vi "Unsubscribe Client.vi"(8 "error in":errorcluster, 9 "Client":string, 10 "Topic Name":string, 11 "Broker in":refnum<class "Broker.lvclass">) -> (0 "error out":errorcluster, 3 "Broker out":refnum<class "Broker.lvclass">)   [LabVIEW 2014, in "Broker.lvclass"]
uses:
  Broker.lvclass
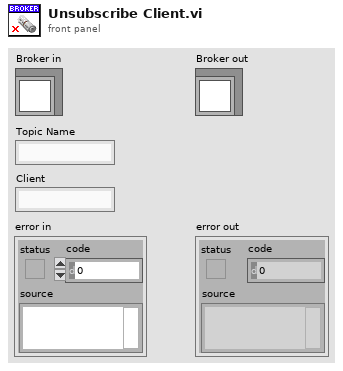
[diagram p1: front panel]
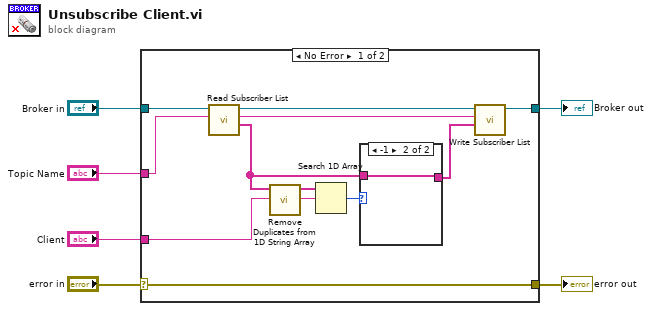
[diagram p0: block diagram]
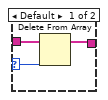
[diagram p2: hidden frame]
diagram:
  n1 = case shown="No Error" "error in" {
    selector: "error in" -> [w16 w23]
    tunnel: [w16 w23] -> w5
    tunnel: [w14 w22] -> w3
    tunnel: "Broker in" -> [w17 w22]
    tunnel: "Topic Name" -> [w13 _]
    tunnel: "Client" -> [w10 _]
    frame No Error {
      n2 = call-dynamic "Read Subscriber List.vi"("Topic Name"=w13, "Broker in"=w17) -> ("Subscriber List"=w8:string[], "Topic Name Out"=w12:string, "Broker out"=w15:refnum<class "Broker.lvclass">)  [unwired: 6 in, 1 out]
      n3 = call "Remove Duplicates from 1D String Array.vi"("Input Array"=w8) -> ("Output Array"=w11:string[])  [unwired: 10 in]
      n4 = Search 1D Array(1D array=w11, element=w10) -> (index of element=w9:i32)  [unwired: 1 in]
      n5 = case shown="-1" w9 {
        selector: w9 -> [w20 _]
        tunnel: w8 -> [w19 w21]
        tunnel: [w18 w21] -> w7
        frame Default {
          n6 = Delete From Array(array=w19, index=w20) -> (array with subset deleted=w18:string[])  [unwired: 1 in, 1 out]
        }
        frame -1 {
        }
      }
      n7 = call-dynamic "Write Subscriber List.vi"("Subscriber List"=w7, "Topic Name"=w12, "Broker in"=w15) -> ("Broker out"=w14:refnum<class "Broker.lvclass">)  [unwired: 7 in, 1 out]
    }
    frame Error {
    }
  }
  "error out" <- w5
  "Broker out" <- w3
